vi "program.vi"() -> ()   [LabVIEW 2020]
uses:
  <vilib>/measure/NI_MABase.lvlib
panel:
  in  "Signal Generator":enum32{"Properties", "Error Cluster/Save"}(tab)
  in  "Type":u16(ring)
  in  "Amplitude":dbl(knob) scale=0.0..50.0
  in  "Frequency":dbl(knob) scale=0.0..10.0 scale format="%#_7g"
  out "AMPL":dbl
  out "FREQ":dbl
  in  "BLOCK":bool
  in  "stop":bool
  in  "SAVE":bool
  out "error out":errorcluster
  out "Waveform Graph":waveform(dbl)(graph)
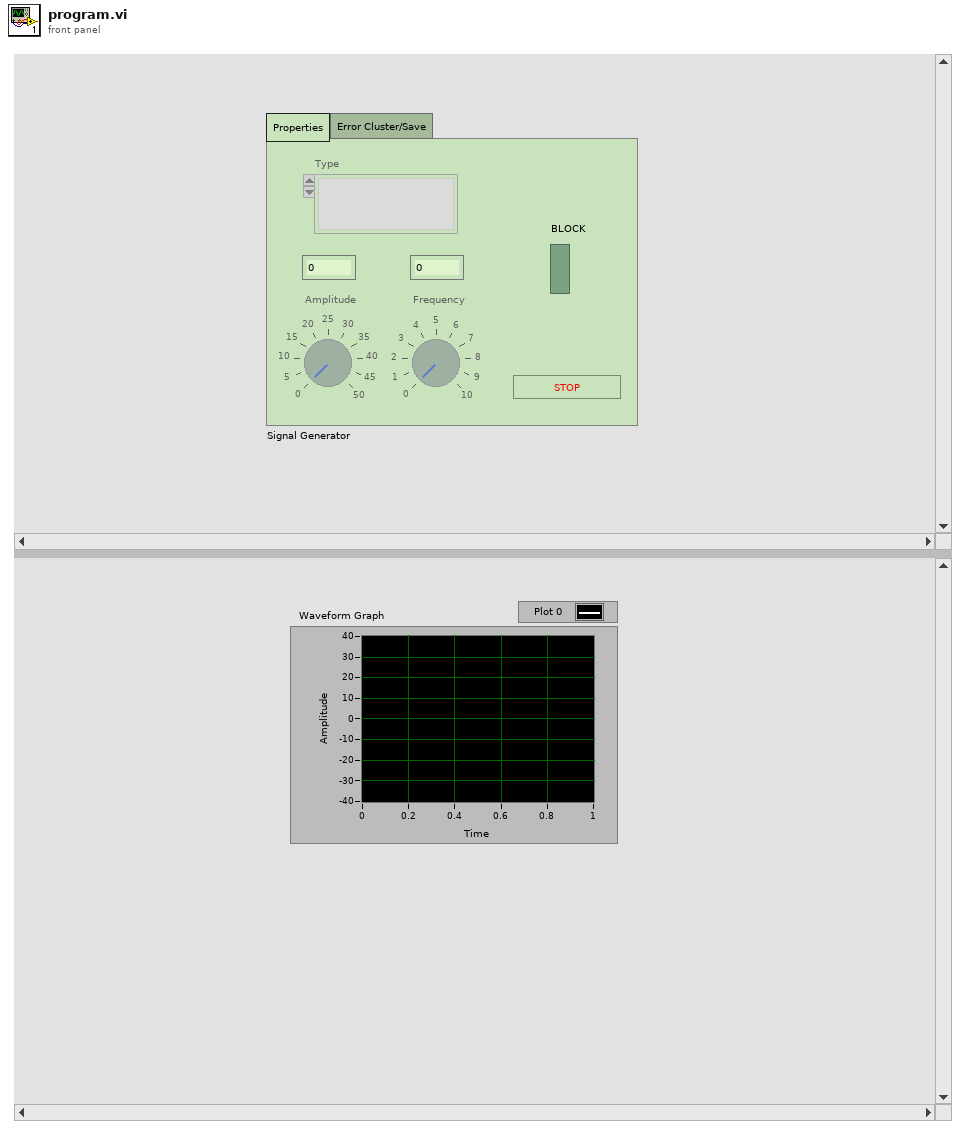
[diagram p1: front panel]
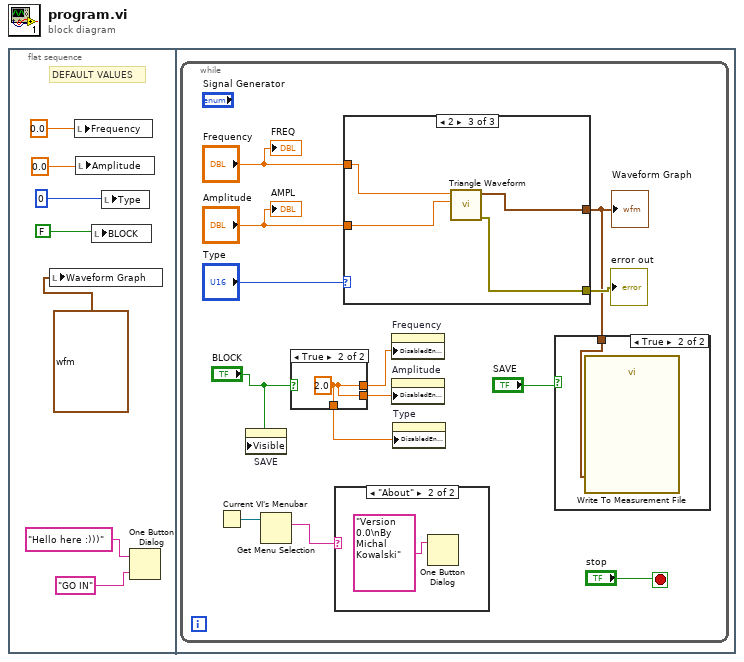
[diagram p0: block diagram]
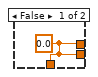
[diagram p4: hidden frame]
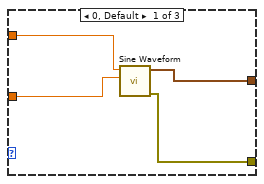
[diagram p5: hidden frame]
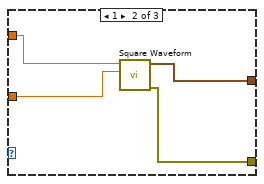
[diagram p6: hidden frame]
diagram:
  n1 = flat-sequence {
    frame #0 {
      # "DEFAULT VALUES"
      n2 = local write "Waveform Graph"(waveform(dbl) {"t0"=timestamp(27.0 s since 1904-01-01), "dt"=0.0, "Y"=array[1000 elements]} ("Waveform Graph")) -> ()
      n3 = local write "Frequency"(0.0) -> ()
      n4 = local write "Amplitude"(0.0) -> ()
      n5 = local write "BLOCK"(FALSE) -> ()
      n6 = local write "Type"(0) -> ()
      n7 = One Button Dialog(message="Hello here :)))", button name ("OK")="GO IN") -> ()  [unwired: 1 out]
    }
    frame #1 {
      n8 = while {
        stop <- "stop" stop-if-true
        n9 = Current VI's Menubar() -> (w9:refnum<k9>)
        n10 = property on="SAVE" class="Bool"("Visible"="BLOCK") -> ()  [unwired: 2 in, 2 out]
        n11 = Get Menu Selection(0:w9) -> (6:w8:string)  [unwired: 3 in, 4 out]
        n12 = case shown="True" "BLOCK" {
          tunnel: [w23 w24] -> w15
          tunnel: [w23 w24] -> w14
          tunnel: [w23 w24] -> w13
          frame False {
            w23 = 0.0
          }
          frame True {
            w24 = 2.0
          }
        }
        n13 = case shown="\"About\"" w8 {
          frame "False", Default {
          }
          frame "About" {
            n14 = One Button Dialog(message="Version 0.0\nBy Michal Kowalski") -> ()  [unwired: 1 in, 1 out]
          }
        }
        n15 = case shown="2" "Type" {
          tunnel: "Amplitude" -> [w28 w31 w35]
          tunnel: "Frequency" -> [w27 w32 w36]
          tunnel: [w26 w30 w34] -> w10
          tunnel: [w25 w29 w33] -> w12
          frame 0, Default {
            n16 = call <vilib>:"Sine Waveform.vi"("amplitude"=w28, "frequency"=w27) -> ("error out"=w25:errorcluster, "signal out"=w26:waveform(dbl))  [unwired: 8 in]
          }
          frame 1 {
            n17 = call <vilib>:"Square Waveform.vi"("amplitude"=w31, "frequency"=w32) -> ("error out"=w29:errorcluster, "signal out"=w30:waveform(dbl))  [unwired: 8 in]
          }
          frame 2 {
            n18 = call <vilib>:"Triangle Waveform.vi"("amplitude"=w35, "frequency"=w36) -> ("error out"=w33:errorcluster, "signal out"=w34:waveform(dbl))  [unwired: 8 in]
          }
        }
        "Waveform Graph" <- w10
        "error out" <- w12
        n19 = property on="Frequency" class="Knob (strict)"("DisabledEnum"=w15) -> ()  [unwired: 2 in, 2 out]
        n20 = property on="Amplitude" class="Knob (strict)"("DisabledEnum"=w14) -> ()  [unwired: 2 in, 2 out]
        n21 = property on="Type" class="Ring (strict)"("DisabledEnum"=w13) -> ()  [unwired: 2 in, 2 out]
        n22 = case shown="True" "SAVE" {
          tunnel: w10 -> [_ w22]
          frame False {
          }
          frame True {
            n23 = call "Write To Measurement File"("Signals"=w22) -> ()  [unwired: 16 in, 3 out]
          }
        }
        "AMPL" <- "Amplitude"
        "FREQ" <- "Frequency"
      }
    }
  }
